vi "NI.History (U64).vi"(1 "value in":u64) -> (0 "Stop?":bool)   [LabVIEW 2020]
doc: "Displays the value of the 32-bit signed integer numeric control and allows conditional breakpoints."
uses:
  <vilib>/Utility/miscctls.llb/LVRowAndColumnUnsignedTypeDef.ctl
panel:
  out "History":i32(listbox)=-1
  in  "Display Style":u16(ring) items=["Decimal", "Hex", "Octal", "Binary", "SI Notation"]
  in  "reset":bool
  # "* Changes to these options take effect the next time the probe runs."
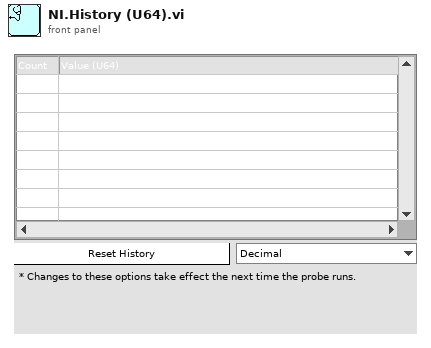
[diagram p1: front panel]
types:
  T1 = typedef "LVRowAndColumnUnsignedTypeDef.ctl" = cluster{"Row":u32, "Column":u32}
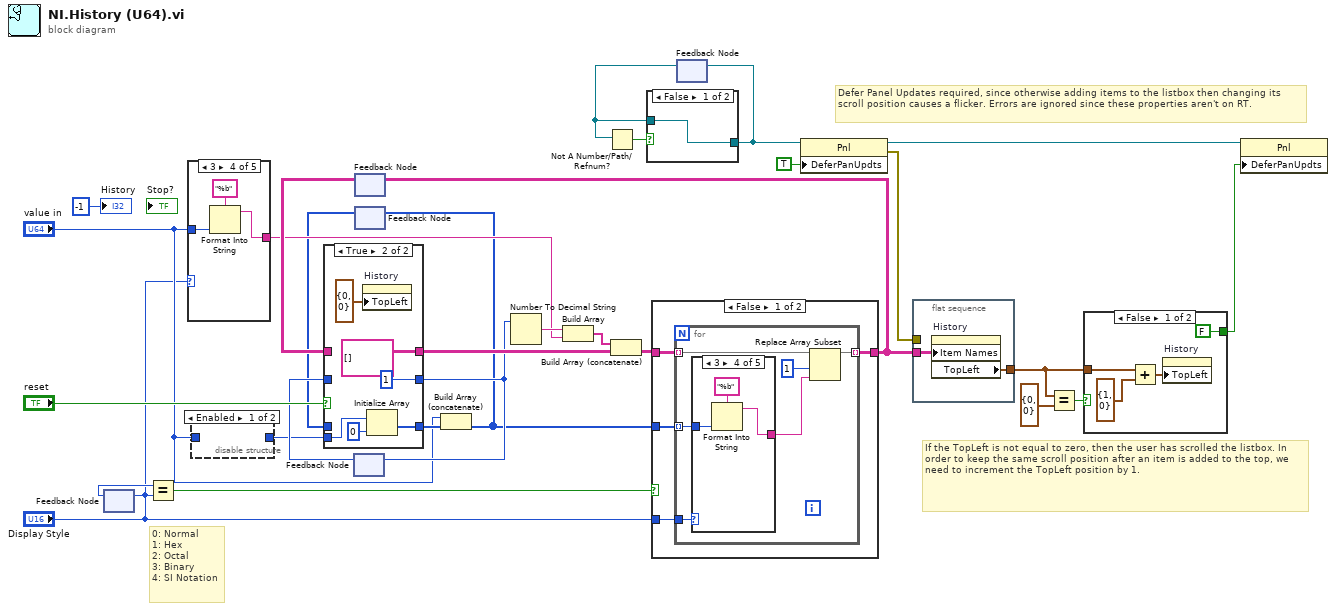
[diagram p0: block diagram]
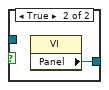
[diagram p3: hidden frame]
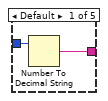
[diagram p5: hidden frame]
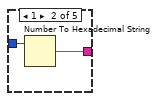
[diagram p6: hidden frame]
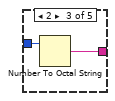
[diagram p7: hidden frame]
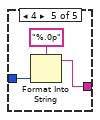
[diagram p8: hidden frame]
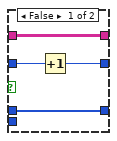
[diagram p9: hidden frame]
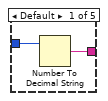
[diagram p10: hidden frame]
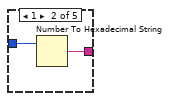
[diagram p11: hidden frame]
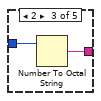
[diagram p12: hidden frame]
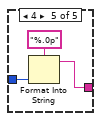
[diagram p13: hidden frame]
diagram:
  # "If the TopLeft is not equal to zero, then the user has scrolled the listbox. In order to keep the same scroll position after an item is added to the top, we need to increment the TopLeft position by 1."
  # "Defer Panel Updates required, since otherwise adding items to the listbox then changing its scroll position causes a flicker. Errors are ignored since these properties aren't on RT."
  # "0: Normal\n1: Hex\n2: Octal\n3: Binary\n4: SI Notation"
  n1 = feedback #1() -> (w12:u16)  [unwired: 1 in]
  n2 = feedback-in #1("Display Style") -> ()
  n3 = Equal?(x=w12, y="Display Style") -> (x = y?=w18:bool)
  n4 = case shown="3" "Display Style" {
    tunnel: "value in" -> [w30 w32 w34 w38 w41]
    tunnel: [w31 w33 w35 w36 w39] -> w19
    frame Default {
      n5 = Number To Decimal String(number=w30) -> (decimal integer string=w31:string)  [unwired: 1 in]
    }
    frame 1 {
      n6 = Number To Hexadecimal String(2:w32) -> (0:w33:string)  [unwired: 1 in]
    }
    frame 2 {
      n7 = Number To Octal String(2:w34) -> (0:w35:string)  [unwired: 1 in]
    }
    frame 3 {
      n8 = Format Into String(format string="%b", w38) -> (resulting string=w36:string)  [unwired: 2 in, 1 out]
    }
    frame 4 {
      n9 = Format Into String(format string="%.0p", w41) -> (resulting string=w39:string)  [unwired: 2 in, 1 out]
    }
  }
  n10 = disable-structure shown="Enabled" {
    disable-tunnel: "value in" -> [_ w42]
    disable-tunnel: [_ w42] -> w17
    frame Enabled {
    }
    frame Disabled {
    }
  }
  n11 = feedback #2() -> (w23:i32)  [unwired: 1 in]
  n12 = feedback #3() -> (w22:string[][])  [unwired: 1 in]
  n13 = feedback #4() -> (w15:u64[])  [unwired: 1 in]
  n14 = case shown="True" "reset" {
    tunnel: w22 -> [w46 _]
    tunnel: w23 -> [w45 _]
    tunnel: [w46 string[][] []] -> w27
    tunnel: [w44 1] -> w24
    tunnel: w17 -> [_ w50]
    tunnel: [w43 w48] -> w16
    tunnel: w15 -> [w43 _]
    frame False {
      n15 = Increment(x=w45) -> (x+1=w44:i32)
    }
    frame True {
      n16 = property on="History" class="MCListbox (strict)"("TopLeft"=T1 {"Row"=0, "Column"=0} ("Top Left Visible Cell")) -> ()  [unwired: 2 in, 2 out]
      n17 = Initialize Array(w50, 0 ("dimension size")) -> (w48:u64[])
    }
  }
  n18 = feedback-in #2(w24) -> ()
  n19 = Build Array (concatenate)("value in", w16) -> (w13:u64[])
  n20 = feedback-in #4(w13) -> ()
  n21 = Number To Decimal String(number=w24) -> (decimal integer string=w25:string)  [unwired: 1 in]
  n22 = Build Array(w25, w19) -> (w26:string[])
  n23 = Build Array (concatenate)(w26, w27) -> (w20:string[][])
  n24 = case shown="False" w18 {
    tunnel: [w55 w75] -> w21
    tunnel: w20 -> [w56 w75]
    tunnel: "Display Style" -> [w54 _]
    tunnel: w13 -> [w53 _]
    frame False {
      n25 = for {
        tunnel: w56 -> [w62] mode=indexing
        tunnel: [w61] -> w55 mode=indexing
        tunnel: w54 -> [w60]
        tunnel: w53 -> [w59] mode=indexing
        n26 = case shown="3" w60 {
          tunnel: w59 -> [w63 w65 w67 w70 w73]
          tunnel: [w64 w66 w68 w69 w72] -> w58
          frame Default {
            n27 = Number To Decimal String(number=w63) -> (decimal integer string=w64:string)  [unwired: 1 in]
          }
          frame 1 {
            n28 = Number To Hexadecimal String(2:w65) -> (0:w66:string)  [unwired: 1 in]
          }
          frame 2 {
            n29 = Number To Octal String(2:w67) -> (0:w68:string)  [unwired: 1 in]
          }
          frame 3 {
            n30 = Format Into String(format string="%b", w70) -> (resulting string=w69:string)  [unwired: 2 in, 1 out]
          }
          frame 4 {
            n31 = Format Into String(format string="%.0p", w73) -> (resulting string=w72:string)  [unwired: 2 in, 1 out]
          }
        }
        n32 = Replace Array Subset(array=w62, new element=w58, index=1) -> (w61:string[])
      }
    }
    frame True {
    }
  }
  n33 = feedback-in #3(w21) -> ()
  n34 = feedback #5() -> (w7:refnum<vi>)  [unwired: 1 in]
  n35 = Not A Number/Path/Refnum?(number/path/refnum=w7) -> (NaN/Path/Refnum?=w8:bool)
  n36 = case shown="False" w8 {
    tunnel: [w76 w77] -> w9
    tunnel: w7 -> [w76 _]
    frame False {
    }
    frame True {
      n37 = property class="VI"() -> ("Panel"=w77:refnum<vi>)  [unwired: 2 in, 2 out]
    }
  }
  n38 = feedback-in #5(w9) -> ()
  n39 = property class="Pnl"(reference=w9, "DeferPanUpdts"=TRUE ("Defer Panel Updates")) -> (reference out=w6:refnum<vi>, error out=w5:errorcluster)  [unwired: 1 in]
  n40 = flat-sequence {
    tunnel: w21 -> [w79]
    tunnel: w5 -> [_]
    tunnel: [w78] -> w2
    frame #0 {
      n41 = property on="History" class="MCListbox (strict)"("Item Names"=w79) -> ("TopLeft"=w78:T1)  [unwired: 2 in, 2 out]
    }
  }
  n42 = Equal?(x=w2, y=T1 {"Row"=0, "Column"=0} ("Top Left Visible Cell")) -> (x = y?=w3:bool)
  n43 = case shown="False" w3 {
    tunnel: w2 -> [w83 _]
    tunnel: [FALSE ("Defer Panel Updates") _] -> w1
    frame False {
      n44 = Add(x=w83, y=T1 {"Row"=1, "Column"=0}) -> (x+y=w81:T1)
      n45 = property on="History" class="MCListbox (strict)"("TopLeft"=w81) -> ()  [unwired: 2 in, 2 out]
    }
    frame True {
    }
  }
  n46 = property class="Pnl"(reference=w6, "DeferPanUpdts"=w1) -> ()  [unwired: 1 in, 2 out]
  "History" <- -1 ("History of Values")
